vi "main_time_control.vi"(9 "Running?":refnum<vi>, 10 "Endtime":refnum<vi>, 11 "Starttime":refnum<vi>) -> ()   [LabVIEW 2019]
uses:
  lib/libSimulationControl/libSimulationControl.lvlib
panel:
  # "*******************************************************************\nBiogas Plant Control\n\nAuthor: Paul Zügel\nGCSC-Frankfurt am Main 2020\n\n*******************************************************************"
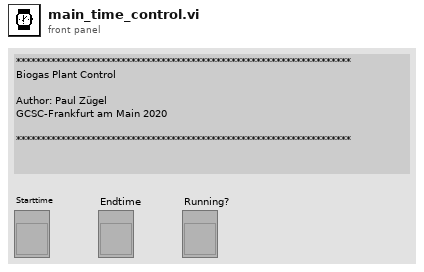
[diagram p1: front panel]
types:
  T1 = enum8{"Enabled", "Disabled", "Disabled and Grayed Out"}
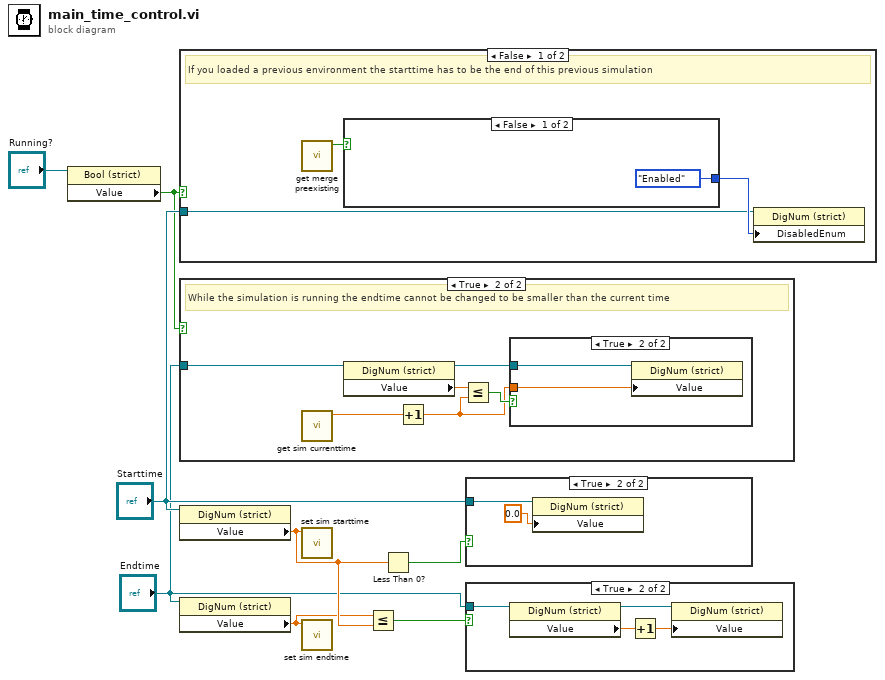
[diagram p0: block diagram]
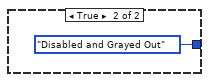
[diagram p4: hidden frame]
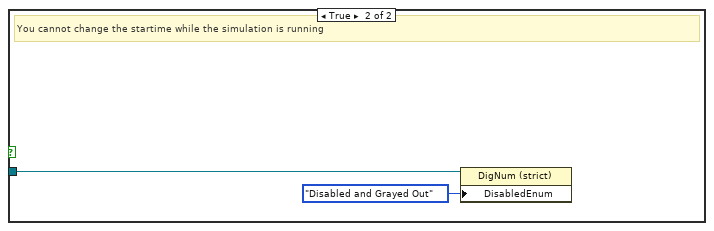
[diagram p5: hidden frame]
diagram:
  n1 = property on="Property Node" class="Bool (strict)"(reference="Running?") -> ("Value"=w2:bool)  [unwired: 1 in, 2 out]
  n2 = case shown="False" w2 {
    tunnel: "Starttime" -> [w10 w14]
    frame False {
      # "If you loaded a previous environment the starttime has to be the end of this previous simulation"
      n3 = call "get merge preexisting.vi"() -> ("function return"=w9:bool)  [unwired: 10 in, 1 out]
      n4 = case shown="False" w9 {
        tunnel: [T1."Enabled" ("Disabled") T1."Disabled and Grayed Out" ("Disabled")] -> w11
        frame False {
        }
        frame True {
        }
      }
      n5 = property class="DigNum (strict)"(reference=w10, "DisabledEnum"=w11) -> ()  [unwired: 1 in, 2 out]
    }
    frame True {
      # "You cannot change the startime while the simulation is running"
      n6 = property class="DigNum (strict)"(reference=w14, "DisabledEnum"=T1."Disabled and Grayed Out" ("Disabled")) -> ()  [unwired: 1 in, 2 out]
    }
  }
  n7 = case shown="True" w2 {
    tunnel: "Endtime" -> [_ w21]
    frame False {
    }
    frame True {
      # "While the simulation is running the endtime cannot be changed to be smaller than the current time"
      n8 = call "get sim currenttime.vi"() -> ("current_time"=w20:dbl)  [unwired: 10 in, 1 out]
      n9 = property class="DigNum (strict)"(reference=w21) -> (reference out=w18:refnum<vi>, "Value"=w19:dbl)  [unwired: 1 in, 1 out]
      n10 = Increment(x=w20) -> (x+1=w16:dbl)
      n11 = Less Or Equal?(x=w19, y=w16) -> (x <= y?=w17:bool)
      n12 = case shown="True" w17 {
        tunnel: w18 -> [_ w23]
        tunnel: w16 -> [_ w22]
        frame False {
        }
        frame True {
          n13 = property class="DigNum (strict)"(reference=w23, "Value"=w22) -> ()  [unwired: 1 in, 2 out]
        }
      }
    }
  }
  n14 = property on="Property Node" class="DigNum (strict)"(reference="Starttime") -> ("Value"=w6:dbl)  [unwired: 1 in, 2 out]
  n15 = property on="Property Node" class="DigNum (strict)"(reference="Endtime") -> ("Value"=w5:dbl)  [unwired: 1 in, 2 out]
  n16 = call "set sim starttime.vi"("time"=w6) -> ()  [unwired: 10 in, 1 out]
  n17 = call "set sim endtime.vi"("time"=w5) -> ()  [unwired: 10 in, 1 out]
  n18 = Less Or Equal?(x=w5, y=w6) -> (x <= y?=w7:bool)
  n19 = Less Than 0?(x=w6) -> (x < 0?=w8:bool)
  n20 = case shown="True" w8 {
    tunnel: "Starttime" -> [_ w24]
    frame False {
    }
    frame True {
      n21 = property on="Property Node" class="DigNum (strict)"(reference=w24, "Value"=0.0 ("Starttime")) -> ()  [unwired: 1 in, 2 out]
    }
  }
  n22 = case shown="True" w7 {
    tunnel: "Endtime" -> [_ w27]
    frame False {
    }
    frame True {
      n23 = property on="Property Node" class="DigNum (strict)"(reference=w27) -> (reference out=w26:refnum<vi>, "Value"=w29:dbl)  [unwired: 1 in, 1 out]
      n24 = Increment(x=w29) -> (x+1=w28:dbl)
      n25 = property on="Property Node" class="DigNum (strict)"(reference=w26, "Value"=w28) -> ()  [unwired: 1 in, 2 out]
    }
  }
